vi "GetProbePlanCoordinates.vi"(8 "Use index as X coord":bool=TRUE, 9 "Probe Card Channels":i32=1) -> (0 "file path":string, 2 "OK?":bool, 3 "Array":T1(array[cluster]))   [LabVIEW 2018] (continued)
328\tX=71372.16\ty=-20769.92 \nLabel=Strip\t329\tX=71025.83\ty=-20682.60 \nLabel=Strip\t330\tX=71379.26\ty=-20613.60 \nLabel=Strip\t331\tX=71032.90\ty=-20526.40 \nLabel=Strip\t332\tX=71386.30\ty=-20457.28 \nLabel=Strip\t333\tX=71039.92\ty=-20370.20 \nLabel=Strip\t334\tX=71393.30\ty=-20300.95 \nLabel=Strip\t335\tX=71046.88\ty=-20213.99 \nLabel=Strip\t336\tX=71400.24\ty=-20144.62 \nLabel=Strip\t337\tX=71053.79\ty=-20057.78 \nLabel=Strip\t338\tX=71407.12\ty=-19988.29 \nLabel=Strip\t339\tX=71060.65\ty=-19901.57 \nLabel=Strip\t340\tX=71413.95\ty=-19831.95 \nLabel=Strip\t341\tX=71067.45\ty=-19745.35 \nLabel=Strip\t342\tX=71420.73\ty=-19675.62 \nLabel=Strip\t343\tX=71074.20\ty=-19589.13 \nLabel=Strip\t344\tX=71427.46\ty=-19519.27 \nLabel=Strip\t345\tX=71080.90\ty=-19432.91 \nLabel=Strip\t346\tX=71434.13\ty=-19362.93 \nLabel=Strip\t347\tX=71087.54\ty=-19276.68 \nLabel=Strip\t348\tX=71440.75\ty=-19206.58 \nLabel=Strip\t349\tX=71094.13\ty=-19120.45 \nLabel=Strip\t350\tX=71447.31\ty=-19050.23 \nLabel=Strip\t351\tX=71100.66\ty=-18964.21 \nLabel=Strip\t352\tX=71453.82\ty=-18893.87 \nLabel=Strip\t353\tX=71107.14\ty=-18807.98 \nLabel=Strip\t354\tX=71460.28\ty=-18737.51 \nLabel=Strip\t355\tX=71113.57\ty=-18651.74 \nLabel=Strip\t356\tX=71466.68\ty=-18581.15 \nLabel=Strip\t357\tX=71119.95\ty=-18495.49 \nLabel=Strip\t358\tX=71473.03\ty=-18424.79 \nLabel=Strip\t359\tX=71126.27\ty=-18339.25 \nLabel=Strip\t360\tX=71479.33\ty=-18268.42 \nLabel=Strip\t361\tX=71132.53\ty=-18183.00 \nLabel=Strip\t362\tX=71485.57\ty=-18112.05 \nLabel=Strip\t363\tX=71138.75\ty=-18026.75 \nLabel=Strip\t364\tX=71491.76\ty=-17955.67 \nLabel=Strip\t365\tX=71144.91\ty=-17870.49 \nLabel=Strip\t366\tX=71497.90\ty=-17799.29 \nLabel=Strip\t367\tX=71151.01\ty=-17714.23 \nLabel=Strip\t368\tX=71503.98\ty=-17642.91 \nLabel=Strip\t369\tX=71157.07\ty=-17557.97 \nLabel=Strip\t370\tX=71510.01\ty=-17486.49 \nLabel=Strip\t371\tX=71163.07\ty=-17401.70 \nLabel=Strip\t372\tX=71515.98\ty=-17330.14 \nLabel=Strip\t373\tX=71169.01\ty=-17245.43 \nLabel=Strip\t374\tX=71521.90\ty=-17173.75 \nLabel=Strip\t375\tX=71174.90\ty=-17089.16 \nLabel=Strip\t376\tX=71527.77\ty=-17017.36 \nLabel=Strip\t377\tX=71180.74\ty=-16932.89 \nLabel=Strip\t378\tX=71533.59\ty=-16860.96 \nLabel=Strip\t379\tX=71186.53\ty=-16776.61 \nLabel=Strip\t380\tX=71539.35\ty=-16704.56 \nLabel=Strip\t381\tX=71192.26\ty=-16620.33 \nLabel=Strip\t382\tX=71545.05\ty=-16548.16 \nLabel=Strip\t383\tX=71197.94\ty=-16464.05 \nLabel=Strip\t384\tX=71550.71\ty=-16391.76 \nLabel=Strip\t385\tX=71203.56\ty=-16307.76 \nLabel=Strip\t386\tX=71556.30\ty=-16235.35 \nLabel=Strip\t387\tX=71209.13\ty=-16151.47 \nLabel=Strip\t388\tX=71561.85\ty=-16078.94 \nLabel=Strip\t389\tX=71214.65\ty=-15995.18 \nLabel=Strip\t390\tX=71567.34\ty=-15922.52 \nLabel=Strip\t391\tX=71220.11\ty=-15838.88 \nLabel=Strip\t392\tX=71572.78\ty=-15766.10 \nLabel=Strip\t393\tX=71225.52\ty=-15682.58 \nLabel=Strip\t394\tX=71578.16\ty=-15609.68 \nLabel=Strip\t395\tX=71230.88\ty=-15526.28 \nLabel=Strip\t396\tX=71583.50\ty=-15453.26 \nLabel=Strip\t397\tX=71236.18\ty=-15369.98 \nLabel=Strip\t398\tX=71588.77\ty=-15296.84 \nLabel=Strip\t399\tX=71241.43\ty=-15213.67 \nLabel=Strip\t400\tX=71594.00\ty=-15140.41 \nLabel=Strip\t401\tX=71246.62\ty=-15057.36 \nLabel=Strip\t402\tX=71599.17\ty=-14983.98 \nLabel=Strip\t403\tX=71251.76\ty=-14901.05 \nLabel=Strip\t404\tX=71604.28\ty=-14827.54 \nLabel=Strip\t405\tX=71256.85\ty=-14744.73 \nLabel=Strip\t406\tX=71609.34\ty=-14671.11 \nLabel=Strip\t407\tX=71261.88\ty=-14588.42 \nLabel=Strip\t408\tX=71614.35\ty=-14514.67 \nLabel=Strip\t409\tX=71266.86\ty=-14432.09 \nLabel=Strip\t410\tX=71619.31\ty=-14358.22 \nLabel=Strip\t411\tX=71271.79\ty=-14275.77 \nLabel=Strip\t412\tX=71624.21\ty=-14201.78 \nLabel=Strip\t413\tX=71276.67\ty=-14119.44 \nLabel=Strip\t414\tX=71629.06\ty=-14045.33 \nLabel=Strip\t415\tX=71281.48\ty=-13963.12 \nLabel=Strip\t416\tX=71633.85\ty=-13888.88 \nLabel=Strip\t417\tX=71286.25\ty=-13806.78 \nLabel=Strip\t418\tX=71638.59\ty=-13732.43 \nLabel=Strip\t419\tX=71290.96\ty=-13650.45 \nLabel=Strip\t420\tX=71643.28\ty=-13575.97 \nLabel=Strip\t421\tX=71295.62\ty=-13494.11 \nLabel=Strip\t422\tX=71647.91\ty=-13419.51 \nLabel=Strip\t423\tX=71300.23\ty=-13337.77 \nLabel=Strip\t424\tX=71652.49\ty=-13263.05 \nLabel=Strip\t425\tX=71304.78\ty=-13181.43 \nLabel=Strip\t426\tX=71657.02\ty=-13106.59 \nLabel=Strip\t427\tX=71309.28\ty=-13025.09 \nLabel=Strip\t428\tX=71661.49\ty=-12950.12 \nLabel=Strip\t429\tX=71313.72\ty=-12868.74 \nLabel=Strip\t430\tX=71665.91\ty=-12793.65 \nLabel=Strip\t431\tX=71318.11\ty=-12712.39 \nLabel=Strip\t432\tX=71670.27\ty=-12637.18 \nLabel=Strip\t433\tX=71322.45\ty=-12556.04 \nLabel=Strip\t434\tX=71674.59\ty=-12480.71 \nLabel=Strip\t435\tX=71326.73\ty=-12399.68 \nLabel=Strip\t436\tX=71678.84\ty=-12324.23 \nLabel=Strip\t437\tX=71330.96\ty=-12243.32 \nLabel=Strip\t438\tX=71683.05\ty=-12167.75 \nLabel=Strip\t439\tX=71335.14\ty=-12086.96 \nLabel=Strip\t440\tX=71687.20\ty=-12011.27 \nLabel=Strip\t441\tX=71339.26\ty=-11930.60 \nLabel=Strip\t442\tX=71691.29\ty=-11854.79 \nLabel=Strip\t443\tX=71343.33\ty=-11774.24 \nLabel=Strip\t444\tX=71695.34\ty=-11698.30 \nLabel=Strip\t445\tX=71347.34\ty=-11617.87 \nLabel=Strip\t446\tX=71699.33\ty=-11541.81 \nLabel=Strip\t447\tX=71351.31\ty=-11461.50 \nLabel=Strip\t448\tX=71703.26\ty=-11385.32 \nLabel=Strip\t449\tX=71355.21\ty=-11305.13 \nLabel=Strip\t450\tX=71707.14\ty=-11228.83 \nLabel=Strip\t451\tX=71359.07\ty=-11148.75 \nLabel=Strip\t452\tX=71710.97\ty=-11072.33 \nLabel=Strip\t453\tX=71362.87\ty=-10992.38 \nLabel=Strip\t454\tX=71714.74\ty=-10915.83 \nLabel=Strip\t455\tX=71366.62\ty=-10836.00 \nLabel=Strip\t456\tX=71718.56\ty=-10734.81 \nLabel=Strip\t457\tX=71370.38\ty=-10660.23 \nLabel=Strip\t458\tX=71722.19\ty=-10588.10 \nLabel=Strip\t459\tX=71373.98\ty=-10513.52 \nLabel=Strip\t460\tX=71725.76\ty=-10441.38 \nLabel=Strip\t461\tX=71377.53\ty=-10366.80 \nLabel=Strip\t462\tX=71729.29\ty=-10294.67 \nLabel=Strip\t463\tX=71381.03\ty=-10220.08 \nLabel=Strip\t464\tX=71732.76\ty=-10147.95 \nLabel=Strip\t465\tX=71384.48\ty=-10073.36 \nLabel=Strip\t466\tX=71736.19\ty=-10001.22 \nLabel=Strip\t467\tX=71387.97\ty=-9897.67 \nLabel=Strip\t468\tX=71739.66\ty=-9820.28 \nLabel=Strip\t469\tX=71391.34\ty=-9741.28 \nLabel=Strip\t470\tX=71743.01\ty=-9663.77 \nLabel=Strip\t471\tX=71394.66\ty=-9584.88 \nLabel=Strip\t472\tX=71746.30\ty=-9507.25 \nLabel=Strip\t473\tX=71397.92\ty=-9428.48 \nLabel=Strip\t474\tX=71749.53\ty=-9350.73 \nLabel=Strip\t475\tX=71401.13\ty=-9272.08 \nLabel=Strip\t476\tX=71752.72\ty=-9194.21 \nLabel=Strip\t477\tX=71404.29\ty=-9115.68 \nLabel=Strip\t478\tX=71755.85\ty=-9037.68 \nLabel=Strip\t479\tX=71407.39\ty=-8959.27 \nLabel=Strip\t480\tX=71758.92\ty=-8881.15 \nLabel=Strip\t481\tX=71410.44\ty=-8802.87 \nLabel=Strip\t482\tX=71761.95\ty=-8724.62 \nLabel=Strip\t483\tX=71413.44\ty=-8646.46 \nLabel=Strip\t484\tX=71764.91\ty=-8568.09 \nLabel=Strip\t485\tX=71416.38\ty=-8490.04 \nLabel=Strip\t486\tX=71767.83\ty=-8411.56 \nLabel=Strip\t487\tX=71419.27\ty=-8333.63 \nLabel=Strip\t488\tX=71770.69\ty=-8255.03 \nLabel=Strip\t489\tX=71422.10\ty=-8177.21 \nLabel=Strip\t490\tX=71773.50\ty=-8098.49 \nLabel=Strip\t491\tX=71424.88\ty=-8020.80 \nLabel=Strip\t492\tX=71776.25\ty=-7941.95 \nLabel=Strip\t493\tX=71427.61\ty=-7864.38 \nLabel=Strip\t494\tX=71778.95\ty=-7785.41 \nLabel=Strip\t495\tX=71430.28\ty=-7707.96 \nLabel=Strip\t496\tX=71781.60\ty=-7628.87 \nLabel=Strip\t497\tX=71432.90\ty=-7551.53 \nLabel=Strip\t498\tX=71784.19\ty=-7472.32 \nLabel=Strip\t499\tX=71435.47\ty=-7395.11 \nLabel=Strip\t500\tX=71786.73\ty=-7315.77 \nLabel=Strip\t501\tX=71437.98\ty=-7238.68 \nLabel=Strip\t502\tX=71789.21\ty=-7159.23 \nLabel=Strip\t503\tX=71440.44\ty=-7082.25 \nLabel=Strip\t504\tX=71791.64\ty=-7002.68 \nLabel=Strip\t505\tX=71442.84\ty=-6925.82 \nLabel=Strip\t506\tX=71794.02\ty=-6846.12 \nLabel=Strip\t507\tX=71445.19\ty=-6769.38 \nLabel=Strip\t508\tX=71796.35\ty=-6689.57 \nLabel=Strip\t509\tX=71447.49\ty=-6612.95 \nLabel=Strip\t510\tX=71798.62\ty=-6533.01 \nLabel=Strip\t511\tX=71449.74\ty=-6456.51 \nLabel=Strip\t512\tX=71800.83\ty=-6376.45 \nLabel=Strip\t513\tX=71451.93\ty=-6300.07 \nLabel=Strip\t514\tX=71803.00\ty=-6219.89 \nLabel=Strip\t515\tX=71454.06\ty=-6143.63 \nLabel=Strip\t516\tX=71805.10\ty=-6063.33 \nLabel=Strip\t517\tX=71456.15\ty=-5987.19 \nLabel=Strip\t518\tX=71807.16\ty=-5906.77 \nLabel=Strip\t519\tX=71458.17\ty=-5830.75 \nLabel=Strip\t520\tX=71809.16\ty=-5750.20 \nLabel=Strip\t521\tX=71460.15\ty=-5674.30 \nLabel=Strip\t522\tX=71811.11\ty=-5593.64 \nLabel=Strip\t523\tX=71462.07\ty=-5517.85 \nLabel=Strip\t524\tX=71813.00\ty=-5437.07 \nLabel=Strip\t525\tX=71463.94\ty=-5361.40 \nLabel=Strip\t526\tX=71814.84\ty=-5280.50 \nLabel=Strip\t527\tX=71465.75\ty=-5204.95 \nLabel=Strip\t528\tX=71816.63\ty=-5123.93 \nLabel=Strip\t529\tX=71467.51\ty=-5048.50 \nLabel=Strip\t530\tX=71818.36\ty=-4967.35 \nLabel=Strip\t531\tX=71469.22\ty=-4892.05 \nLabel=Strip\t532\tX=71820.04\ty=-4810.78 \nLabel=Strip\t533\tX=71470.87\ty=-4735.59 \nLabel=Strip\t534\tX=71821.67\ty=-4654.20 \nLabel=Strip\t535\tX=71472.47\ty=-4579.14 \nLabel=Strip\t536\tX=71823.24\ty=-4497.62 \nLabel=Strip\t537\tX=71474.02\ty=-4422.68 \nLabel=Strip\t538\tX=71824.75\ty=-4341.04 \nLabel=Strip\t539\tX=71475.51\ty=-4266.22 \nLabel=Strip\t540\tX=71826.22\ty=-4184.46 \nLabel=Strip\t541\tX=71476.95\ty=-4109.75 \nLabel=Strip\t542\tX=71827.63\ty=-4027.88 \nLabel=Strip\t543\tX=71478.33\ty=-3953.29 \nLabel=Strip\t544\tX=71828.98\ty=-3871.30 \nLabel=Strip\t545\tX=71479.66\ty=-3796.83 \nLabel=Strip\t546\tX=71830.29\ty=-3714.71 \nLabel=Strip\t547\tX=71480.94\ty=-3640.36 \nLabel=Strip\t548\tX=71831.54\ty=-3558.12 \nLabel=Strip\t549\tX=71482.16\ty=-3483.89 \nLabel=Strip\t550\tX=71832.73\ty=-3401.54 \nLabel=Strip\t551\tX=71483.33\ty=-3327.42 \nLabel=Strip\t552\tX=71833.87\ty=-3244.89 \nLabel=Strip\t553\tX=71484.45\ty=-3170.95 \nLabel=Strip\t554\tX=71834.96\ty=-3088.35 \nLabel=Strip\t555\tX=71485.51\ty=-3014.48 \nLabel=Strip\t556\tX=71835.99\ty=-2931.76 \nLabel=Strip\t557\tX=71486.52\ty=-2858.01 \nLabel=Strip\t558\tX=71836.97\ty=-2775.17 \nLabel=Strip\t559\tX=71487.47\ty=-2701.53 \nLabel=Strip\t560\tX=71837.90\ty=-2618.57 \nLabel=Strip\t561\tX=71488.38\ty=-2545.06 \nLabel=Strip\t562\tX=71838.77\ty=-2461.97 \nLabel=Strip\t563\tX=71489.22\ty=-2388.58 \nLabel=Strip\t564\tX=71839.59\ty=-2305.37 \nLabel=Strip\t565\tX=71490.02\ty=-2232.10 \nLabel=Strip\t566\tX=71840.36\ty=-2148.77 \nLabel=Strip\t567\tX=71490.76\ty=-2075.62 \nLabel=Strip\t568\tX=71841.07\ty=-1992.17 \nLabel=Strip\t569\tX=71491.44\ty=-1919.14 \nLabel=Strip\t570\tX=71841.72\ty=-1835.57 \nLabel=Strip\t571\tX=71492.07\ty=-1762.65 \nLabel=Strip\t572\tX=71842.33\ty=-1678.97 \nLabel=Strip\t573\tX=71492.65\ty=-1606.17 \nLabel=Strip\t574\tX=71842.88\ty=-1522.36 \nLabel=Strip\t575\tX=71493.18\ty=-1449.69 \nLabel=Strip\t576\tX=71843.37\ty=-1365.76 \nLabel=Strip\t577\tX=71493.65\ty=-1293.20 \nLabel=Strip\t578\tX=71843.82\ty=-1209.15 \nLabel=Strip\t579\tX=71494.07\ty=-1136.71 \nLabel=Strip\t580\tX=71844.20\ty=-1052.54 \nLabel=Strip\t581\tX=71494.43\ty=-980.22 \nLabel=Strip\t582\tX=71844.54\ty=-895.93 \nLabel=Strip\t583\tX=71494.74\ty=-823.73 \nLabel=Strip\t584\tX=71844.82\ty=-739.32 \nLabel=Strip\t585\tX=71495.00\ty=-667.24 \nLabel=Strip\t586\tX=71845.05\ty=-582.71 \nLabel=Strip\t587\tX=71495.20\ty=-510.75 \nLabel=Strip\t588\tX=71845.22\ty=-426.10 \nLabel=Strip\t589\tX=71495.35\ty=-354.26 \nLabel=Strip\t590\tX=71845.34\ty=-269.48 \nLabel=Strip\t591\tX=71495.44\ty=-197.76 \nLabel=Strip\t592\tX=71845.41\ty=-112.87 \nLabel=Strip\t593\tX=71495.48\ty=-41.27 \nLabel=Strip\t594\tX=71845.42\ty=43.75 \nLabel=Strip\t595\tX=71495.47\ty=115.23 \nLabel=Strip\t596\tX=71845.38\ty=200.36 \nLabel=Strip\t597\tX=71495.40\ty=271.73 \nLabel=Strip\t598\tX=71845.28\ty=356.98 \nLabel=Strip\t599\tX=71495.28\ty=428.22 \nLabel=Strip\t600\tX=71845.13\ty=513.60 \nLabel=Strip\t601\tX=71495.11\ty=584.72 \nLabel=Strip\t602\tX=71844.93\ty=670.22 \nLabel=Strip\t603\tX=71494.88\ty=741.22 \nLabel=Strip\t604\tX=71844.67\ty=826.84 \nLabel=Strip\t605\tX=71494.60\ty=897.73 \nLabel=Strip\t606\tX=71844.36\ty=983.46 \nLabel=Strip\t607\tX=71494.27\ty=1054.23 \nLabel=Strip\t608\tX=71844.00\ty=1140.09 \nLabel=Strip\t609\tX=71493.88\ty=1210.73 \nLabel=Strip\t610\tX=71843.58\ty=1296.71 \nLabel=Strip\t611\tX=71493.43\ty=1367.24 \nLabel=Strip\t612\tX=71843.10\ty=1453.34 \nLabel=Strip\t613\tX=71492.94\ty=1523.74 \nLabel=Strip\t614\tX=71842.58\ty=1609.96 \nLabel=Strip\t615\tX=71492.39\ty=1680.25 \nLabel=Strip\t616\tX=71842.00\ty=1766.59 \nLabel=Strip\t617\tX=71491.78\ty=1836.75 \nLabel=Strip\t618\tX=71841.37\ty=1923.21 \nLabel=Strip\t619\tX=71491.13\ty=1993.26 \nLabel=Strip\t620\tX=71840.68\ty=2079.84 \nLabel=Strip\t621\tX=71490.42\ty=2149.77 \nLabel=Strip\t622\tX=71839.94\ty=2236.47 \nLabel=Strip\t623\tX=71489.65\ty=2306.28 \nLabel=Strip\t624\tX=71839.14\ty=2393.10 \nLabel=Strip\t625\tX=71488.83\ty=2462.79 \nLabel=Strip\t626\tX=71838.29\ty=2549.73 \nLabel=Strip\t627\tX=71487.96\ty=2619.30 \nLabel=Strip\t628\tX=71837.39\ty=2706.36 \nLabel=Strip\t629\tX=71487.03\ty=2775.81 \nLabel=Strip\t630\tX=71836.43\ty=2862.99 \nLabel=Strip\t631\tX=71486.05\ty=2932.32 \nLabel=Strip\t632\tX=71835.42\ty=3019.63 \nLabel=Strip\t633\tX=71485.02\ty=3088.83 \nLabel=Strip\t634\tX=71834.36\ty=3176.26 \nLabel=Strip\t635\tX=71483.93\ty=3245.35 \nLabel=Strip\t636\tX=71833.24\ty=3332.89 \nLabel=Strip\t637\tX=71482.79\ty=3401.86 \nLabel=Strip\t638\tX=71832.07\ty=3489.53 \nLabel=Strip\t639\tX=71481.59\ty=3558.37 \nLabel=Strip\t640\tX=71830.84\ty=3646.16 \nLabel=Strip\t641\tX=71480.34\ty=3714.89 \nLabel=Strip\t642\tX=71829.57\ty=3802.80 \nLabel=Strip\t643\tX=71479.04\ty=3871.24 \nLabel=Strip\t644\tX=71828.23\ty=3959.43 \nLabel=Strip\t645\tX=71477.68\ty=4027.92 \nLabel=Strip\t646\tX=71826.85\ty=4116.07 \nLabel=Strip\t647\tX=71476.27\ty=4184.44 \nLabel=Strip\t648\tX=71825.40\ty=4272.71 \nLabel=Strip\t649\tX=71474.81\ty=4340.96 \nLabel=Strip\t650\tX=71823.91\ty=4429.35 \nLabel=Strip\t651\tX=71473.29\ty=4497.47 \nLabel=Strip\t652\tX=71822.36\ty=4585.98 \nLabel=Strip\t653\tX=71471.72\ty=4653.99 \nLabel=Strip\t654\tX=71820.76\ty=4742.62 \nLabel=Strip\t655\tX=71470.09\ty=4810.51 \nLabel=Strip\t656\tX=71819.10\ty=4899.26 \nLabel=Strip\t657\tX=71468.41\ty=4967.03 \nLabel=Strip\t658\tX=71817.39\ty=5055.90 \nLabel=Strip\t659\tX=71466.68\ty=5123.55 \nLabel=Strip\t660\tX=71815.63\ty=5212.54 \nLabel=Strip\t661\tX=71464.89\ty=5280.07 \nLabel=Strip\t662\tX=71813.81\ty=5369.18 \nLabel=Strip\t663\tX=71463.05\ty=5436.59 \nLabel=Strip\t664\tX=71811.94\ty=5525.82 \nLabel=Strip\t665\tX=71461.16\ty=5593.11 \nLabel=Strip\t666\tX=71810.02\ty=5682.47 \nLabel=Strip\t667\tX=71459.21\ty=5749.64 \nLabel=Strip\t668\tX=71808.04\ty=5839.11 \nLabel=Strip\t669\tX=71457.21\ty=5906.16 \nLabel=Strip\t670\tX=71806.00\ty=5995.75 \nLabel=Strip\t671\tX=71455.15\ty=6062.68 \nLabel=Strip\t672\tX=71803.92\ty=6152.39 \nLabel=Strip\t673\tX=71453.04\ty=6219.20 \nLabel=Strip\t674\tX=71801.78\ty=6309.04 \nLabel=Strip\t675\tX=71450.88\ty=6375.72 \nLabel=Strip\t676\tX=71799.58\ty=6465.68 \nLabel=Strip\t677\tX=71448.66\ty=6532.25 \nLabel=Strip\t678\tX=71797.34\ty=6622.32 \nLabel=Strip\t679\tX=71446.39\ty=6688.77 \nLabel=Strip\t680\tX=71795.03\ty=6778.97 \nLabel=Strip\t681\tX=71444.07\ty=6845.29 \nLabel=Strip\t682\tX=71792.68\ty=6935.61 \nLabel=Strip\t683\tX=71441.69\ty=7001.82 \nLabel=Strip\t684\tX=71790.27\ty=7092.25 \nLabel=Strip\t685\tX=71439.26\ty=7158.34 \nLabel=Strip\t686\tX=71787.80\ty=7248.90 \nLabel=Strip\t687\tX=71436.77\ty=7314.87 \nLabel=Strip\t688\tX=71785.29\ty=7405.54 \nLabel=Strip\t689\tX=71434.23\ty=7471.39 \nLabel=Strip\t690\tX=71782.72\ty=7562.19 \nLabel=Strip\t691\tX=71431.64\ty=7627.92 \nLabel=Strip\t692\tX=71780.09\ty=7718.83 \nLabel=Strip\t693\tX=71428.99\ty=7784.44 \nLabel=Strip\t694\tX=71777.41\ty=7875.48 \nLabel=Strip\t695\tX=71426.29\ty=7940.97 \nLabel=Strip\t696\tX=71774.68\ty=8032.12 \nLabel=Strip\t697\tX=71423.53\ty=8097.49 \nLabel=Strip\t698\tX=71771.89\ty=8188.77 \nLabel=Strip\t699\tX=71420.72\ty=8254.01 \nLabel=Strip\t700\tX=71769.05\ty=8345.41 \nLabel=Strip\t701\tX=71417.86\ty=8410.54 \nLabel=Strip\t702\tX=71766.16\ty=8502.06 \nLabel=Strip\t703\tX=71414.95\ty=8567.07 \nLabel=Strip\t704\tX=71763.21\ty=8658.70 \nLabel=Strip\t705\tX=71411.97\ty=8723.59 \nLabel=Strip\t706\tX=71760.21\ty=8815.35 \nLabel=Strip\t707\tX=71408.95\ty=8880.12 \nLabel=Strip\t708\tX=71757.15\ty=8971.99 \nLabel=Strip\t709\tX=71405.87\ty=9036.64 \nLabel=Strip\t710\tX=71754.04\ty=9128.64 \nLabel=Strip\t711\tX=71402.74\ty=9193.17 \nLabel=Strip\t712\tX=71750.88\ty=9285.28 \nLabel=Strip\t713\tX=71399.56\ty=9349.69 \nLabel=Strip\t714\tX=71747.66\ty=9441.93 \nLabel=Strip\t715\tX=71396.32\ty=9506.22 \nLabel=Strip\t716\tX=71744.39\ty=9598.57 \nLabel=Strip\t717\tX=71393.02\ty=9662.74 \nLabel=Strip\t718\tX=71741.07\ty=9755.22 \nLabel=Strip\t719\tX=71389.68\ty=9819.26 \nLabel=Strip\t720\tX=71737.69\ty=9911.86 \nLabel=Strip\t721\tX=71386.28\ty=9975.79 \nLabel=Strip\t722\tX=71734.26\ty=10068.51 \nLabel=Strip\t723\tX=71382.82\ty=10132.31 \nLabel=Strip\t724\tX=71730.77\ty=10225.15 \nLabel=Strip\t725\tX=71379.31\ty=10288.84 \nLabel=Strip\t726\tX=71727.23\ty=10381.79 \nLabel=Strip\t727\tX=71375.75\ty=10445.36 \nLabel=Strip\t728\tX=71723.64\ty=10538.44 \nLabel=Strip\t729\tX=71372.13\ty=10601.89 \nLabel=Strip\t730\tX=71719.99\ty=10695.08 \nLabel=Strip\t731\tX=71368.47\ty=10758.41 \nLabel=Strip\t732\tX=71716.29\ty=10851.73 \nLabel=Strip\t733\tX=71364.74\ty=10914.93 \nLabel=Strip\t734\tX=71712.53\ty=11008.37 \nLabel=Strip\t735\tX=71360.97\ty=11071.46 \nLabel=Strip\t736\tX=71708.72\ty=11165.01 \nLabel=Strip\t737\tX=71357.13\ty=11227.98 \nLabel=Strip\t738\tX=71704.86\ty=11321.66 \nLabel=Strip\t739\tX=71353.25\ty=11384.50 \nLabel=Strip\t740\tX=71700.94\ty=11478.30 \nLabel=Strip\t741\tX=71349.31\ty=11541.02 \nLabel=Strip\t742\tX=71696.97\ty=11634.94 \nLabel=Strip\t743\tX=71345.32\ty=11697.55 \nLabel=Strip\t744\tX=71692.94\ty=11791.58 \nLabel=Strip\t745\tX=71341.27\ty=11854.07 \nLabel=Strip\t746\tX=71688.87\ty=11948.22 \nLabel=Strip\t747\tX=71337.17\ty=12010.59 \nLabel=Strip\t748\tX=71684.73\ty=12104.86 \nLabel=Strip\t749\tX=71333.02\ty=12167.11 \nLabel=Strip\t750\tX=71680.55\ty=12261.51 \nLabel=Strip\t751\tX=71328.81\ty=12323.63 \nLabel=Strip\t752\tX=71676.31\ty=12418.15 \nLabel=Strip\t753\tX=71324.55\ty=12480.15 \nLabel=Strip\t754\tX=71672.01\ty=12574.79 \nLabel=Strip\t755\tX=71320.23\ty=12636.67 \nLabel=Strip\t756\tX=71667.67\ty=12731.43 \nLabel=Strip\t757\tX=71315.86\ty=12793.19 \nLabel=Strip\t758\tX=71663.26\ty=12888.06 \nLabel=Strip\t759\tX=71311.44\ty=12949.71 \nLabel=Strip\t760\tX=71658.81\ty=13044.70 \nLabel=Strip\t761\tX=71306.96\ty=13106.23 \nLabel=Strip\t762\tX=71654.30\ty=13201.34 \nLabel=Strip\t763\tX=71302.43\ty=13262.74 \nLabel=Strip\t764\tX=71649.73\ty=13357.98 \nLabel=Strip\t765\tX=71297.85\ty=13419.26 \nLabel=Strip\t766\tX=71645.12\ty=13514.62 \nLabel=Strip\t767\tX=71293.21\ty=13575.78 \nLabel=Strip\t768\tX=71640.45\ty=13671.25 \nLabel=Strip\t769\tX=71288.52\ty=13732.29 \nLabel=Strip\t770\tX=71635.72\ty=13827.89 \nLabel=Strip\t771\tX=71283.77\ty=13888.81 \nLabel=Strip\t772\tX=71630.94\ty=13984.52 \nLabel=Strip\t773\tX=71278.97\ty=14045.32 \nLabel=Strip\t774\tX=71626.11\ty=14141.16 \nLabel=Strip\t775\tX=71274.12\ty=14201.84 \nLabel=Strip\t776\tX=71621.22\ty=14297.79 \nLabel=Strip\t777\tX=71269.21\ty=14358.35 \nLabel=Strip\t778\tX=71616.28\ty=14454.42 \nLabel=Strip\t779\tX=71264.25\ty=14514.86 \nLabel=Strip\t780\tX=71611.29\ty=14611.06 \nLabel=Strip\t781\tX=71259.23\ty=14671.38 \nLabel=Strip\t782\tX=71606.24\ty=14767.69 \nLabel=Strip\t783\tX=71254.17\ty=14827.89 \nLabel=Strip\t784\tX=71601.14\ty=14924.32 \nLabel=Strip\t785\tX=71249.04\ty=14984.40 \nLabel=Strip\t786\tX=71595.98\ty=15080.95 \nLabel=Strip\t787\tX=71243.87\ty=15140.91 \nLabel=Strip\t788\tX=71590.77\ty=15237.58 \nLabel=Strip\t789\tX=71238.64\ty=15297.42 \nLabel=Strip\t790\tX=71585.51\ty=15394.21 \nLabel=Strip\t791\tX=71233.35\ty=15453.93 \nLabel=Strip\t792\tX=71580.19\ty=15550.84 \nLabel=Strip\t793\tX=71228.01\ty=15610.44 \nLabel=Strip\t794\tX=71574.82\ty=15707.46 \nLabel=Strip\t795\tX=71222.62\ty=15766.94 \nLabel=Strip\t796\tX=71569.40\ty=15864.09 \nLabel=Strip\t797\tX=71217.18\ty=15923.45 \nLabel=Strip\t798\tX=71563.92\ty=16020.72 \nLabel=Strip\t799\tX=71211.68\ty=16079.95 \nLabel=Strip\t800\tX=71558.38\ty=16177.34 \nLabel=Strip\t801\tX=71206.12\ty=16236.46 \nLabel=Strip\t802\tX=71552.80\ty=16333.97 \nLabel=Strip\t803\tX=71200.52\ty=16392.96 \nLabel=Strip\t804\tX=71547.16\ty=16490.59 \nLabel=Strip\t805\tX=71194.86\ty=16549.46 \nLabel=Strip\t806\tX=71541.46\ty=16647.21 \nLabel=Strip\t807\tX=71189.14\ty=16705.97 \nLabel=Strip\t808\tX=71535.71\ty=16803.83 \nLabel=Strip\t809\tX=71183.37\ty=16862.47 \nLabel=Strip\t810\tX=71529.91\ty=16960.45 \nLabel=Strip\t811\tX=71177.55\ty=17018.97 \nLabel=Strip\t812\tX=71524.05\ty=17117.07 \nLabel=Strip\t813\tX=71171.67\ty=17175.46 \nLabel=Strip\t814\tX=71518.14\ty=17273.69 \nLabel=Strip\t815\tX=71165.74\ty=17331.96 \nLabel=Strip\t816\tX=71512.18\ty=17430.31 \nLabel=Strip\t817\tX=71159.76\ty=17488.46 \nLabel=Strip\t818\tX=71506.16\ty=17586.92 \nLabel=Strip\t819\tX=71153.72\ty=17644.96 \nLabel=Strip\t820\tX=71500.09\ty=17743.54 \nLabel=Strip\t821\tX=71147.63\ty=17801.45 \nLabel=Strip\t822\tX=71493.97\ty=17900.15 \nLabel=Strip\t823\tX=71141.48\ty=17957.94 \nLabel=Strip\t824\tX=71487.79\ty=18056.77 \nLabel=Strip\t825\tX=71135.29\ty=18114.44 \nLabel=Strip\t826\tX=71481.55\ty=18213.38 \nLabel=Strip\t827\tX=71129.03\ty=18270.93 \nLabel=Strip\t828\tX=71475.27\ty=18369.99 \nLabel=Strip\t829\tX=71122.73\ty=18427.42 \nLabel=Strip\t830\tX=71468.93\ty=18526.60 \nLabel=Strip\t831\tX=71116.37\ty=18583.91 \nLabel=Strip\t832\tX=71462.53\ty=18683.21 \nLabel=Strip\t833\tX=71109.95\ty=18740.39 \nLabel=Strip\t834\tX=71456.08\ty=18839.81 \nLabel=Strip\t835\tX=71103.48\ty=18896.88 \nLabel=Strip\t836\tX=71449.58\ty=18996.42 \nLabel=Strip\t837\tX=71096.96\ty=19053.37 \nLabel=Strip\t838\tX=71443.02\ty=19153.03 \nLabel=Strip\t839\tX=71090.38\ty=19209.85 \nLabel=Strip\t840\tX=71436.41\ty=19309.63 \nLabel=Strip\t841\tX=71083.75\ty=19366.34 \nLabel=Strip\t842\tX=71429.75\ty=19466.23 \nLabel=Strip\t843\tX=71077.07\ty=19522.82 \nLabel=Strip\t844\tX=71423.03\ty=19622.83 \nLabel=Strip\t845\tX=71070.33\ty=19679.30 \nLabel=Strip\t846\tX=71416.26\ty=19779.43 \nLabel=Strip\t847\tX=71063.54\ty=19835.78 \nLabel=Strip\t848\tX=71409.43\ty=19936.03 \nLabel=Strip\t849\tX=71056.70\ty=19992.25 \nLabel=Strip\t850\tX=71402.55\ty=20092.63 \nLabel=Strip\t851\tX=71049.80\ty=20148.73 \nLabel=Strip\t852\tX=71395.62\ty=20249.22 \nLabel=Strip\t853\tX=71042.85\ty=20305.21 \nLabel=Strip\t854\tX=71388.63\ty=20405.82 \nLabel=Strip\t855\tX=71035.84\ty=20461.68 \nLabel=Strip\t856\tX=71381.59\ty=20562.41 \nLabel=Strip\t857\tX=71028.78\ty=20618.15 \nLabel=Strip\t858\tX=71374.50\ty=20719.00 \nLabel=Strip\t859\tX=71021.66\ty=20774.63 \nLabel=Strip\t860\tX=71367.35\ty=20875.59 \nLabel=Strip\t861\tX=71014.50\ty=20931.09 \nLabel=Strip\t862\tX=71360.14\ty=21032.18 \nLabel=Strip\t863\tX=71007.27\ty=21087.56 \nLabel=Strip\t864\tX=71352.89\ty=21188.77 \nLabel=Strip\t865\tX=71000.00\ty=21244.03 \nLabel=Strip\t866\tX=71345.58\ty=21345.36 \nLabel=Strip\t867\tX=70992.67\ty=21400.50 \nLabel=Strip\t868\tX=71338.21\ty=21501.94 \nLabel=Strip\t869\tX=70985.28\ty=21556.96 \nLabel=Strip\t870\tX=71330.79\ty=21658.52 \nLabel=Strip\t871\tX=70977.85\ty=21713.42 \nLabel=Strip\t872\tX=71323.32\ty=21815.11 \nLabel=Strip\t873\tX=70970.36\ty=21869.88 \nLabel=Strip\t874\tX=71315.80\ty=21971.69 \nLabel=Strip\t875\tX=70962.81\ty=22026.34 \nLabel=Strip\t876\tX=71308.21\ty=22128.26 \nLabel=Strip\t877\tX=70955.21\ty=22182.80 \nLabel=Strip\t878\tX=71300.58\ty=22284.84 \nLabel=Strip\t879\tX=70947.56\ty=22339.26 \nLabel=Strip\t880\tX=71292.89\ty=22441.42 \nLabel=Strip\t881\tX=70939.85\ty=22495.71 \nLabel=Strip\t882\tX=71285.15\ty=22597.99 \nLabel=Strip\t883\tX=70932.09\ty=22652.16 \nLabel=Strip\t884\tX=71277.36\ty=22754.56 \nLabel=Strip\t885\tX=70924.28\ty=22808.61 \nLabel=Strip\t886\tX=71269.51\ty=22911.13 \nLabel=Strip\t887\tX=70916.41\ty=22965.06 \nLabel=Strip\t888\tX=71261.60\ty=23067.70 \nLabel=Strip\t889\tX=70908.49\ty=23121.51 \nLabel=Strip\t890\tX=71253.65\ty=23224.27 \nLabel=Strip\t891\tX=70900.51\ty=23277.96 \nLabel=Strip\t892\tX=71245.63\ty=23380.83 \nLabel=Strip\t893\tX=70892.48\ty=23434.40 \nLabel=Strip\t894\tX=71237.57\ty=23537.40 \nLabel=Strip\t895\tX=70884.40\ty=23590.85 \nLabel=Strip\t896\tX=71229.45\ty=23693.96 \nLabel=Strip\t897\tX=70876.26\ty=23747.29 \nLabel=Strip\t898\tX=71221.28\ty=23850.52 \nLabel=Strip\t899\tX=70868.07\ty=23903.73 \nLabel=Strip\t900\tX=71213.05\ty=24007.08 \nLabel=Strip\t901\tX=70859.83\ty=24060.16 \nLabel=Strip\t902\tX=71204.77\ty=24163.63 \nLabel=Strip\t903\tX=70851.53\ty=24216.60 \nLabel=Strip\t904\tX=71196.44\ty=24320.19 \nLabel=Strip\t905\tX=70843.18\ty=24373.03 \nLabel=Strip\t906\tX=71188.05\ty=24476.74 \nLabel=Strip\t907\tX=70834.77\ty=24529.46 \nLabel=Strip\t908\tX=71179.61\ty=24633.29 \nLabel=Strip\t909\tX=70826.31\ty=24685.89 \nLabel=Strip\t910\tX=71171.11\ty=24789.84 \nLabel=Strip\t911\tX=70817.79\ty=24842.32 \nLabel=Strip\t912\tX=71162.56\ty=24946.39 \nLabel=Strip\t913\tX=70809.23\ty=24998.75 \nLabel=Strip\t914\tX=71153.96\ty=25102.93 \nLabel=Strip\t915\tX=70800.60\ty=25155.17 \nLabel=Strip\t916\tX=71145.30\ty=25259.48 \nLabel=Strip\t917\tX=70791.93\ty=25311.60 \nLabel=Strip\t918\tX=71136.59\ty=25416.02 \nLabel=Strip\t919\tX=70783.20\ty=25468.02 \nLabel=Strip\t920\tX=71127.82\ty=25572.56 \nLabel=Strip\t921\tX=70774.42\ty=25624.43 \nLabel=Strip\t922\tX=71119.00\ty=25729.09 \nLabel=Strip\t923\tX=70765.58\ty=25780.85 \nLabel=Strip\t924\tX=71110.13\ty=25885.63 \nLabel=Strip\t925\tX=70756.69\ty=25937.27 \nLabel=Strip\t926\tX=71101.20\ty=26042.16 \nLabel=Strip\t927\tX=70747.74\ty=26093.68 \nLabel=Strip\t928\tX=71092.22\ty=26198.69 \nLabel=Strip\t929\tX=70738.74\ty=26250.09 \nLabel=Strip\t930\tX=71083.19\ty=26355.22 \nLabel=Strip\t931\tX=70729.69\ty=26406.50 \nLabel=Strip\t932\tX=71074.10\ty=26511.75 \nLabel=Strip\t933\tX=70720.59\ty=26562.90 \nLabel=Strip\t934\tX=71064.96\ty=26668.27 \nLabel=Strip\t935\tX=70711.43\ty=26719.31 \nLabel=Strip\t936\tX=71055.76\ty=26824.80 \nLabel=Strip\t937\tX=70702.21\ty=26875.71 \nLabel=Strip\t938\tX=71046.51\ty=26981.32 \nLabel=Strip\t939\tX=70692.94\ty=27032.11 \nLabel=Strip\t940\tX=71037.21\ty=27137.84 \nLabel=Strip\t941\tX=70683.62\ty=27188.51 \nLabel=Strip\t942\tX=71027.85\ty=27294.35 \nLabel=Strip\t943\tX=70674.25\ty=27344.90 \nLabel=Strip\t944\tX=71018.44\ty=27450.87 \nLabel=Strip\t945\tX=70664.82\ty=27501.29 \nLabel=Strip\t946\tX=71008.97\ty=27607.38 \nLabel=Strip\t947\tX=70655.33\ty=27657.69 \nLabel=Strip\t948\tX=70999.45\ty=27763.89 \nLabel=Strip\t949\tX=70645.80\ty=27814.07 \nLabel=Strip\t950\tX=70989.88\ty=27920.40 \nLabel=Strip\t951\tX=70636.21\ty=27970.46 \nLabel=Strip\t952\tX=70980.25\ty=28076.90 \nLabel=Strip\t953\tX=70626.56\ty=28126.84 \nLabel=Strip\t954\tX=70970.57\ty=28233.40 \nLabel=Strip\t955\tX=70616.86\ty=28283.23 \nLabel=Strip\t956\tX=70960.83\ty=28389.90 \nLabel=Strip\t957\tX=70607.11\ty=28439.61 \nLabel=Strip\t958\tX=70951.04\ty=28546.40 \nLabel=Strip\t959\tX=70597.30\ty=28595.98 \nLabel=Strip\t960\tX=70941.20\ty=28702.90 \nLabel=Strip\t961\tX=70587.44\ty=28752.36 \nLabel=Strip\t962\tX=70931.30\ty=28859.39 \nLabel=Strip\t963\tX=70577.53\ty=28908.73 \nLabel=Strip\t964\tX=70921.35\ty=29015.88 \nLabel=Strip\t965\tX=70567.56\ty=29065.10 \nLabel=Strip\t966\tX=70911.35\ty=29172.37 \nLabel=Strip\t967\tX=70557.54\ty=29221.47 \nLabel=Strip\t968\tX=70901.29\ty=29328.86 \nLabel=Strip\t969\tX=70547.47\ty=29377.83 \nLabel=Strip\t970\tX=70891.18\ty=29485.34 \nLabel=Strip\t971\tX=70537.34\ty=29534.20 \nLabel=Strip\t972\tX=70881.01\ty=29641.82 \nLabel=Strip\t973\tX=70527.15\ty=29690.56 \nLabel=Strip\t974\tX=70870.79\ty=29798.30 \nLabel=Strip\t975\tX=70516.92\ty=29846.92 \nLabel=Strip\t976\tX=70860.52\ty=29954.78 \nLabel=Strip\t977\tX=70506.63\ty=30003.27 \nLabel=Strip\t978\tX=70850.19\ty=30111.25 \nLabel=Strip\t979\tX=70496.28\ty=30159.62 \nLabel=Strip\t980\tX=70839.81\ty=30267.72 \nLabel=Strip\t981\tX=70485.88\ty=30315.97 \nLabel=Strip\t982\tX=70829.37\ty=30424.19 \nLabel=Strip\t983\tX=70475.43\ty=30472.32 \nLabel=Strip\t984\tX=70818.88\ty=30580.66 \nLabel=Strip\t985\tX=70464.92\ty=30628.67 \nLabel=Strip\t986\tX=70808.34\ty=30737.12 \nLabel=Strip\t987\tX=70454.37\ty=30785.01 \nLabel=Strip\t988\tX=70797.74\ty=30893.59 \nLabel=Strip\t989\tX=70443.75\ty=30941.35 \nLabel=Strip\t990\tX=70787.09\ty=31050.04 \nLabel=Strip\t991\tX=70433.08\ty=31097.69 \nLabel=Strip\t992\tX=70776.39\ty=31206.50 \nLabel=Strip\t993\tX=70422.36\ty=31254.02 \nLabel=Strip\t994\tX=70765.63\ty=31362.95 \nLabel=Strip\t995\tX=70411.59\ty=31410.35 \nLabel=Strip\t996\tX=70754.81\ty=31519.40 \nLabel=Strip\t997\tX=70400.76\ty=31566.68 \nLabel=Strip\t998\tX=70743.95\ty=31675.85 \nLabel=Strip\t999\tX=70389.88\ty=31723.01 \nLabel=Strip\t1000\tX=70733.03\ty=31832.30 \nLabel=Strip\t1001\tX=70378.94\ty=31879.34 \nLabel=Strip\t1002\tX=70722.05\ty=31988.74 \nLabel=Strip\t1003\tX=70367.95\ty=32035.66 \nLabel=Strip\t1004\tX=70711.02\ty=32145.18 \nLabel=Strip\t1005\tX=70356.90\ty=32191.98 \nLabel=Strip\t1006\tX=70699.94\ty=32301.61 \nLabel=Strip\t1007\tX=70345.81\ty=32348.29 \nLabel=Strip\t1008\tX=70688.81\ty=32458.05 \nLabel=Strip\t1009\tX=70334.65\ty=32504.60 \nLabel=Strip\t1010\tX=70677.62\ty=32614.48 \nLabel=Strip\t1011\tX=70323.45\ty=32660.91 \nLabel=Strip\t1012\tX=70666.37\ty=32770.91 \nLabel=Strip\t1013\tX=70312.19\ty=32817.22 \nLabel=Strip\t1014\tX=70655.07\ty=32927.33 \nLabel=Strip\t1015\tX=70300.87\ty=32973.53 \nLabel=Strip\t1016\tX=70643.72\ty=33083.76 \nLabel=Strip\t1017\tX=70289.51\ty=33129.83 \nLabel=Strip\t1018\tX=70632.32\ty=33240.18 \nLabel=Strip\t1019\tX=70278.09\ty=33286.13 \nLabel=Strip\t1020\tX=70620.86\ty=33396.59 \nLabel=Strip\t1021\tX=70266.61\ty=33442.42 \nLabel=Strip\t1022\tX=70609.35\ty=33553.01 \nLabel=Strip\t1023\tX=70255.08\ty=33598.71 \nLabel=Strip\t1024\tX=70597.78\ty=33709.42 \nLabel=Strip\t1025\tX=70243.50\ty=33755.00 \nLabel=Strip\t1026\tX=70586.16\ty=33865.83 \nLabel=Strip\t1027\tX=70231.86\ty=33911.29 \nLabel=Strip\t1028\tX=70574.48\ty=34022.29 \nLabel=Strip\t1029\tX=70220.17\ty=34067.57 \nLabel=Strip\t1030\tX=70562.75\ty=34178.63 \nLabel=Strip\t1031\tX=70208.43\ty=34223.86 \nLabel=Strip\t1032\tX=70550.97\ty=34335.03 \nLabel=Strip\t1033\tX=70196.63\ty=34380.13 \nLabel=Strip\t1034\tX=70539.14\ty=34491.43 \nLabel=Strip\t1035\tX=70184.78\ty=34536.41 \nLabel=Strip\t1036\tX=70527.25\ty=34647.82 \nLabel=Strip\t1037\tX=70172.87\ty=34692.68 \nLabel=Strip\t1038\tX=70515.30\ty=34804.21 \nLabel=Strip\t1039\tX=70160.91\ty=34848.95 \nLabel=Strip\t1040\tX=70503.30\ty=34960.60 \nLabel=Strip\t1041\tX=70148.90\ty=35005.21 \nLabel=Strip\t1042\tX=70491.25\ty=35116.98 \nLabel=Strip\t1043\tX=70136.83\ty=35161.48 \nLabel=Strip\t1044\tX=70479.15\ty=35273.36 \nLabel=Strip\t1045\tX=70124.71\ty=35317.74 \nLabel=Strip\t1046\tX=70466.99\ty=35429.74 \nLabel=Strip\t1047\tX=70112.54\ty=35473.99 \nLabel=Strip\t1048\tX=70454.77\ty=35586.11 \nLabel=Strip\t1049\tX=70100.31\ty=35630.25 \nLabel=Strip\t1050\tX=70442.51\ty=35742.49 \nLabel=Strip\t1051\tX=70088.02\ty=35786.50 \nLabel=Strip\t1052\tX=70430.18\ty=35898.85 \nLabel=Strip\t1053\tX=70075.69\ty=35942.74 \nLabel=Strip\t1054\tX=70417.81\ty=36055.22 \nLabel=Strip\t1055\tX=70063.30\ty=36098.99 \nLabel=Strip\t1056\tX=70405.38\ty=36211.58 \nLabel=Strip\t1057\tX=70050.85\ty=36255.23 \nLabel=Strip\t1058\tX=70392.90\ty=36367.94 \nLabel=Strip\t1059\tX=70038.36\ty=36411.46 \nLabel=Strip\t1060\tX=70380.36\ty=36524.29 \nLabel=Strip\t1061\tX=70025.80\ty=36567.70 \nLabel=Strip\t1062\tX=70367.77\ty=36680.64 \nLabel=Strip\t1063\tX=70013.20\ty=36723.93 \nLabel=Strip\t1064\tX=70355.13\ty=36836.99 \nLabel=Strip\t1065\tX=70000.54\ty=36880.15 \nLabel=Strip\t1066\tX=70342.43\ty=36993.34 \nLabel=Strip\t1067\tX=69987.83\ty=37036.38 \nLabel=Strip\t1068\tX=70329.68\ty=37149.68 \nLabel=Strip\t1069\tX=69975.06\ty=37192.60 \nLabel=Strip\t1070\tX=70316.87\ty=37306.02 \nLabel=Strip\t1071\tX=69962.24\ty=37348.81 \nLabel=Strip\t1072\tX=70304.01\ty=37462.35 \nLabel=Strip\t1073\tX=69949.36\ty=37505.03 \nLabel=Strip\t1074\tX=70291.10\ty=37618.68 \nLabel=Strip\t1075\tX=69936.44\ty=37661.24 \nLabel=Strip\t1076\tX=70278.13\ty=37775.01 \nLabel=Strip\t1077\tX=69923.45\ty=37817.45 \nLabel=Strip\t1078\tX=70265.11\ty=37931.34 \nLabel=Strip\t1079\tX=69910.42\ty=37973.65 \nLabel=Strip\t1080\tX=70252.03\ty=38087.66 \nLabel=Strip\t1081\tX=69897.33\ty=38129.85 \nLabel=Strip\t1082\tX=70238.90\ty=38243.97 \nLabel=Strip\t1083\tX=69884.18\ty=38286.05 \nLabel=Strip\t1084\tX=70225.72\ty=38400.29 \nLabel=Strip\t1085\tX=69870.99\ty=38442.24 \nLabel=Strip\t1086\tX=70212.48\ty=38556.60 \nLabel=Strip\t1087\tX=69857.74\ty=38598.43 \nLabel=Strip\t1088\tX=70199.19\ty=38712.91 \nLabel=Strip\t1089\tX=69844.43\ty=38754.61 \nLabel=Strip\t1090\tX=70185.85\ty=38869.21 \nLabel=Strip\t1091\tX=69831.07\ty=38910.80 \nLabel=Strip\t1092\tX=70172.45\ty=39025.51 \nLabel=Strip\t1093\tX=69817.66\ty=39066.97 \nLabel=Strip\t1094\tX=70159.00\ty=39181.81 \nLabel=Strip\t1095\tX=69804.19\ty=39223.15 \nLabel=Strip\t1096\tX=70145.49\ty=39338.10 \nLabel=Strip\t1097\tX=69790.67\ty=39379.32 \nLabel=Strip\t1098\tX=70131.93\ty=39494.39 \nLabel=Strip\t1099\tX=69777.10\ty=39535.49 \nLabel=Strip\t1100\tX=70118.32\ty=39650.67 \nLabel=Strip\t1101\tX=69763.47\ty=39691.65 \nLabel=Strip\t1102\tX=70104.65\ty=39806.95 \nLabel=Strip\t1103\tX=69749.79\ty=39847.81 \nLabel=Strip\t1104\tX=70090.93\ty=39963.23 \nLabel=Strip\t1105\tX=69736.05\ty=40003.97 \nLabel=Strip\t1106\tX=70077.15\ty=40119.51 \nLabel=Strip\t1107\tX=69722.26\ty=40160.12 \nLabel=Strip\t1108\tX=70063.32\ty=40275.78 \nLabel=Strip\t1109\tX=69708.42\ty=40316.27 \nLabel=Strip\t1110\tX=70049.44\ty=40432.05 \nLabel=Strip\t1111\tX=69694.52\ty=40472.42 \nLabel=Strip\t1112\tX=70035.50\ty=40588.31 \nLabel=Strip\t1113\tX=69680.57\ty=40628.56 \nLabel=Strip\t1114\tX=70021.51\ty=40744.57 \nLabel=Strip\t1115\tX=69666.57\ty=40784.70 \nLabel=Strip\t1116\tX=70007.47\ty=40900.82 \nLabel=Strip\t1117\tX=69652.51\ty=40940.83 \nLabel=Strip\t1118\tX=69993.36\ty=41057.16 \nLabel=Strip\t1119\tX=69638.40\ty=41096.96 \nLabel=Strip\t1120\tX=69979.22\ty=41213.32 \nLabel=Strip\t1121\tX=69624.23\ty=41253.09 \nLabel=Strip\t1122\tX=69965.01\ty=41369.57 \nLabel=Strip\t1123\tX=69610.01\ty=41409.21 \nLabel=Strip\t1124\tX=69950.75\ty=41525.81 \nLabel=Strip\t1125\tX=69595.74\ty=41565.33 \nLabel=Strip\t1126\tX=69936.44\ty=41682.04 \nLabel=Strip\t1127\tX=69581.41\ty=41721.44 \nLabel=Strip\t1128\tX=69922.07\ty=41838.28 \nLabel=Strip\t1129\tX=69567.03\ty=41877.56 \nLabel=Strip\t1130\tX=69907.65\ty=41994.50 \nLabel=Strip\t1131\tX=69552.59\ty=42033.66 \nLabel=Strip\t1132\tX=69893.17\ty=42150.73 \nLabel=Strip\t1133\tX=69538.10\ty=42189.77 \nLabel=Strip\t1134\tX=69878.64\ty=42306.95 \nLabel=Strip\t1135\tX=69523.56\ty=42345.87 \nLabel=Strip\t1136\tX=69864.06\ty=42463.17 \nLabel=Strip\t1137\tX=69508.96\ty=42501.96 \nLabel=Strip\t1138\tX=69849.42\ty=42619.38 \nLabel=Strip\t1139\tX=69494.31\ty=42658.05 \nLabel=Strip\t1140\tX=69834.73\ty=42775.59 \nLabel=Strip\t1141\tX=69479.61\ty=42814.14 \nLabel=Strip\t1142\tX=69819.99\ty=42931.79 \nLabel=Strip\t1143\tX=69464.85\ty=42970.22 \nLabel=Strip\t1144\tX=69805.19\ty=43087.99 \nLabel=Strip\t1145\tX=69450.04\ty=43126.30 \nLabel=Strip\t1146\tX=69790.34\ty=43244.19 \nLabel=Strip\t1147\tX=69435.17\ty=43282.38 \nLabel=Strip\t1148\tX=69775.43\ty=43400.38 \nLabel=Strip\t1149\tX=69420.25\ty=43438.45 \nLabel=Strip\t1150\tX=69760.47\ty=43556.57 \nLabel=Strip\t1151\tX=69405.28\ty=43594.51 \nLabel=Strip\t1152\tX=69745.46\ty=43712.75 \nLabel=Strip\t1153\tX=69390.25\ty=43750.58 \nLabel=Strip\t1154\tX=69730.39\ty=43868.93 \nRegion=Segment\t0B\nLabel=Strip\t1\tX=70381.22\ty=-46341.35 \nLabel=Strip\t2\tX=70737.97\ty=-46292.22 \nLabel=Strip\t3\tX=70397.08\ty=-46185.54 \nLabel=Strip\t4\tX=70753.82\ty=-46136.29 \nLabel=Strip\t5\tX=70412.89\ty=-46029.72 \nLabel=Strip\t6\tX=70769.60\ty=-45980.35 \nLabel=Strip\t7\tX=70428.64\ty=-45873.90 \nLabel=Strip\t8\tX=70785.34\ty=-45824.40 \nLabel=Strip\t9\tX=70444.34\ty=-45718.07 \nLabel=Strip\t10\tX=70801.02\ty=-45668.44 \nLabel=Strip\t11\tX=70459.98\ty=-45562.23 \nLabel=Strip\t12\tX=70816.65\ty=-45512.48 \nLabel=Strip\t13\tX=70475.58\ty=-45406.38 \nLabel=Strip\t14\tX=70832.23\ty=-45356.52 \nLabel=Strip\t15\tX=70491.11\ty=-45250.53 \nLabel=Strip\t16\tX=70847.75\ty=-45200.54 \nLabel=Strip\t17\tX=70506.60\ty=-45094.68 \nLabel=Strip\t18\tX=70863.22\ty=-45044.56 \nLabel=Strip\t19\tX=70522.03\ty=-44938.81 \nLabel=Strip\t20\tX=70878.63\ty=-44888.58 \nLabel=Strip\t21\tX=70537.41\ty=-44782.94 \nLabel=Strip\t22\tX=70893.99\ty=-44732.58 \nLabel=Strip\t23\tX=70552.74\ty=-44627.07 \nLabel=Strip\t24\tX=70909.30\ty=-44576.59 \nLabel=Strip\t25\tX=70568.01\ty=-44471.19 \nLabel=Strip\t26\tX=70924.56\ty=-44420.58 \nLabel=Strip\t27\tX=70583.23\ty=-44315.30 \nLabel=Strip\t28\tX=70939.76\ty=-44264.57 \nLabel=Strip\t29\tX=70598.39\ty=-44159.40 \nLabel=Strip\t30\tX=70954.90\ty=-44108.55 \nLabel=Strip\t31\tX=70613.50\ty=-44003.50 \nLabel=Strip\t32\tX=70970.00\ty=-43952.53 \nLabel=Strip\t33\tX=70628.56\ty=-43847.60 \nLabel=Strip\t34\tX=70985.04\ty=-43796.50 \nLabel=Strip\t35\tX=70643.57\ty=-43691.68 \nLabel=Strip\t36\tX=71000.03\ty=-43640.46 \nLabel=Strip\t37\tX=70658.52\ty=-43535.76 \nLabel=Strip\t38\tX=71014.96\ty=-43484.42 \nLabel=Strip\t39\tX=70673.42\ty=-43379.84 \nLabel=Strip\t40\tX=71029.84\ty=-43328.37 \nLabel=Strip\t41\tX=70688.27\ty=-43223.91 \nLabel=Strip\t42\tX=71044.67\ty=-43172.32 \nLabel=Strip\t43\tX=70703.06\ty=-43067.97 \nLabel=Strip\t44\tX=71059.45\ty=-43016.26 \nLabel=Strip\t45\tX=70717.80\ty=-42912.03 \nLabel=Strip\t46\tX=71074.17\ty=-42860.19 \nLabel=Strip\t47\tX=70732.48\ty=-42756.08 \nLabel=Strip\t48\tX=71088.84\ty=-42704.12 \nLabel=Strip\t49\tX=70747.11\ty=-42600.12 \nLabel=Strip\t50\tX=71103.45\ty=-42548.04 \nLabel=Strip\t51\tX=70761.69\ty=-42444.16 \nLabel=Strip\t52\tX=71118.01\ty=-42391.95 \nLabel=Strip\t53\tX=70776.22\ty=-42288.19 \nLabel=Strip\t54\tX=71132.52\ty=-42235.86 \nLabel=Strip\t55\tX=70790.69\ty=-42132.22 \nLabel=Strip\t56\tX=71146.97\ty=-42079.77 \nLabel=Strip\t57\tX=70805.11\ty=-41976.24 \nLabel=Strip\t58\tX=71161.37\ty=-41923.67 \nLabel=Strip\t59\tX=70819.47\ty=-41820.25 \nLabel=Strip\t60\tX=71175.72\ty=-41767.56 \nLabel=Strip\t61\tX=70833.78\ty=-41664.26 \nLabel=Strip\t62\tX=71190.01\ty=-41611.44 \nLabel=Strip\t63\tX=70848.04\ty=-41508.26 \nLabel=Strip\t64\tX=71204.25\ty=-41455.32 \nLabel=Strip\t65\tX=70862.25\ty=-41352.26 \nLabel=Strip\t66\tX=71218.44\ty=-41299.20 \nLabel=Strip\t67\tX=70876.40\ty=-41196.25 \nLabel=Strip\t68\tX=71232.57\ty=-41143.06 \nLabel=Strip\t69\tX=70890.50\ty=-41040.23 \nLabel=Strip\t70\tX=71246.65\ty=-40986.92 \nLabel=Strip\t71\tX=70904.54\ty=-40884.21 \nLabel=Strip\t72\tX=71260.68\ty=-40830.78 \nLabel=Strip\t73\tX=70918.53\ty=-40728.19 \nLabel=Strip\t74\tX=71274.65\ty=-40674.63 \nLabel=Strip\t75\tX=70932.47\ty=-40572.15 \nLabel=Strip\t76\tX=71288.57\ty=-40518.48 \nLabel=Strip\t77\tX=70946.35\ty=-40416.11 \nLabel=Strip\t78\tX=71302.44\ty=-40362.31 \nLabel=Strip\t79\tX=70960.19\ty=-40260.07 \nLabel=Strip\t80\tX=71316.25\ty=-40206.15 \nLabel=Strip\t81\tX=70973.96\ty=-40104.02 \nLabel=Strip\t82\tX=71330.01\ty=-40049.97 \nLabel=Strip\t83\tX=70987.69\ty=-39947.96 \nLabel=Strip\t84\tX=71343.71\ty=-39893.79 \nLabel=Strip\t85\tX=71001.36\ty=-39791.90 \nLabel=Strip\t86\tX=71357.37\ty=-39737.61 \nLabel=Strip\t87\tX=71014.98\ty=-39635.83 \nLabel=Strip\t88\tX=71370.97\ty=-39581.42 \nLabel=Strip\t89\tX=71028.54\ty=-39479.76 \nLabel=Strip\t90\tX=71384.51\ty=-39425.23 \nLabel=Strip\t91\tX=71042.05\ty=-39323.68 \nLabel=Strip\t92\tX=71398.00\ty=-39269.02 \nLabel=Strip\t93\tX=71055.51\ty=-39167.60 \nLabel=Strip\t94\tX=71411.44\ty=-39112.82 \nLabel=Strip\t95\tX=71068.91\ty=-39011.51 \nLabel=Strip\t96\tX=71424.83\ty=-38956.60 \nLabel=Strip\t97\tX=71082.26\ty=-38855.41 \nLabel=Strip\t98\tX=71438.16\ty=-38800.39 \nLabel=Strip\t99\tX=71095.56\ty=-38699.31 \nLabel=Strip\t100\tX=71451.44\ty=-38644.16 
